vi "Ex7.vi"() -> ()   [LabVIEW 2016]
panel:
  out "?":dbl
  in  "?":dbl
  in  "?":dbl
  # "2"
  # "2"
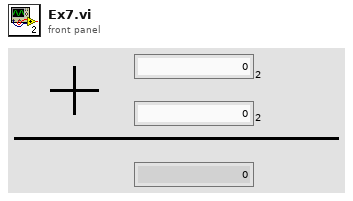
[diagram p1: front panel]
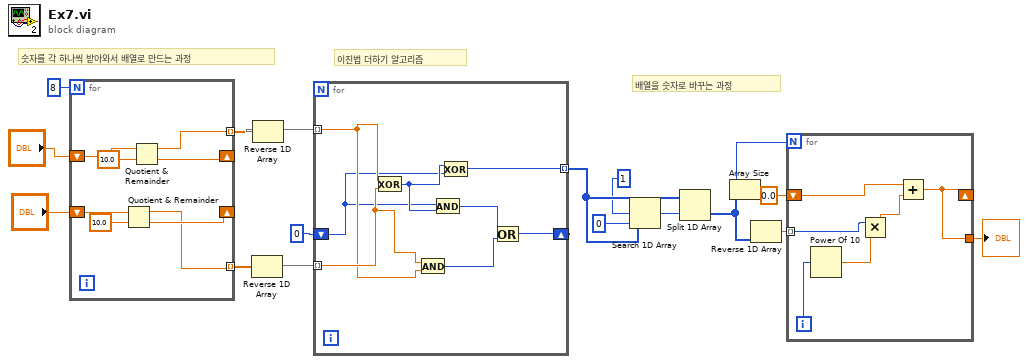
[diagram p0: block diagram]
diagram:
  # "배열을 숫자로 바꾸는 과정"
  # "이진법 더하기 알고리즘"
  # "숫자를 각 하나씩 받아와서 배열로 만드는 과정"
  n1 = for {
    N: 8 -> [_]
    shift-right: [w22] -> _
    shift-left: "?" -> [w25]
    tunnel: [w23] -> w12 mode=indexing
    shift-right: [w19] -> _
    shift-left: "?" -> [w20]
    tunnel: [w18] -> w13 mode=indexing
    n2 = Quotient & Remainder(x=w20, y=10.0) -> (x-y*floor(x/y)=w18:dbl, floor(x/y)=w19:dbl)
    n3 = Quotient & Remainder(x=w25, y=10.0) -> (x-y*floor(x/y)=w23:dbl, floor(x/y)=w22:dbl)
  }
  n4 = Reverse 1D Array(array=w13) -> (reversed array=w11:dbl[])
  n5 = Reverse 1D Array(array=w12) -> (reversed array=w15:dbl[])
  n6 = for {
    tunnel: w15 -> [w29] mode=indexing
    tunnel: w11 -> [w30] mode=indexing
    shift-right: [w27] -> _
    shift-left: 0 ("y") -> [w28]
    tunnel: [w26] -> w7 mode=indexing
    n7 = Exclusive Or(1:w30, 2:w29) -> (0:w33:i32)
    n8 = And(x=w30, y=w29) -> (x .and. y?=w31:i32)
    n9 = And(x=w28, y=w33) -> (x .and. y?=w32:i32)
    n10 = Exclusive Or(1:w28, 2:w33) -> (0:w26:i32)
    n11 = Or(x=w32, y=w31) -> (x .or. y?=w27:i32)
  }
  n12 = Search 1D Array(1D array=w7, element=1 ("원소"), start index (0)=0 ("시작 인덱스(0)")) -> (index of element=w8:i32)
  n13 = Split 1D Array(array=w7, index=w8) -> (second subarray=w5:i32[])  [unwired: 1 out]
  n14 = Array Size(array=w5) -> (size(s)=w6:i32)
  n15 = Reverse 1D Array(array=w5) -> (reversed array=w4:i32[])
  n16 = for {
    N: w6 -> [_]
    tunnel: w4 -> [w38] mode=indexing
    shift-right: [w34] -> _
    shift-left: 0.0 -> [w36]
    tunnel: [w34] -> w3
    i -> [w39]
    n17 = Power Of 10(x=w39) -> (10^x=w37:dbl)
    n18 = Multiply(x=w38, y=w37) -> (x*y=w35:dbl)
    n19 = Add(x=w36, y=w35) -> (x+y=w34:dbl)
  }
  "?" <- w3
